vi "KrakenCommandPower.vi"(0 "Device Reference (in)":T1, 5 "Output Mode":T2(ring), 7 "Control Mode":enum16{"Safety", "Power"}(ring), 9 "Power or Testing Power":dbl, 11 "Error (in)":errorcluster) -> ()   [LabVIEW 2023]
doc: "Wrapper for commanding the power of a Talon FX motor controller. Supports voltage and safety interlock. Also supports the standard actuator testing interface and and the only sending new values on change."
uses:
  <vilib>/Rock Robotics/WPI/ThirdParty/Phoenix6/DeviceReference.ctl
  <vilib>/Rock Robotics/WPI/ThirdParty/Phoenix6/controls/DutyCycleOut SetControl.vi
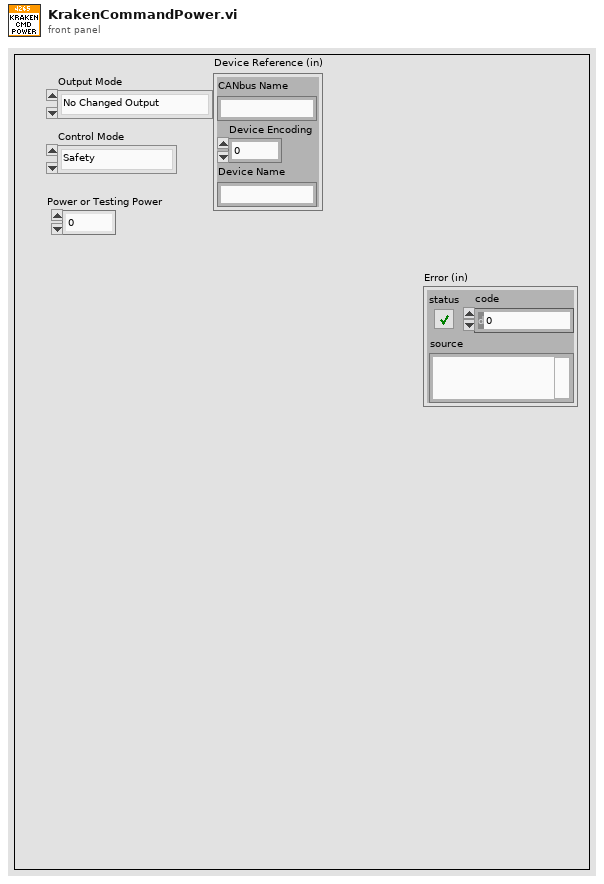
[diagram p1: front panel]
types:
  T1 = typedef "DeviceReference.ctl" = cluster{"CANbus Name":string, "Device Encoding":u32, "Device Name":string}
  T2 = enum16{"No Changed Output", "New Normal Output", "New Testing Output"}
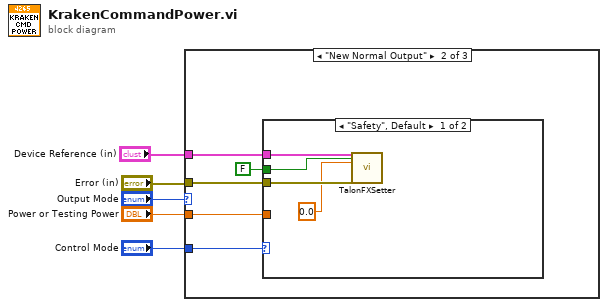
[diagram p0: block diagram]
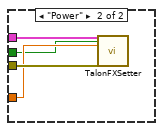
[diagram p3: hidden frame]
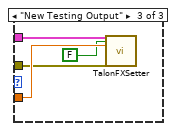
[diagram p4: hidden frame]
diagram:
  n1 = case shown="\"New Normal Output\"" "Output Mode" {
    tunnel: "Power or Testing Power" -> [_ w7 w22]
    tunnel: "Device Reference (in)" -> [_ w10 w20]
    tunnel: "Control Mode" -> [_ w9 _]
    tunnel: "Error (in)" -> [_ w8 w21]
    frame "No Changed Output", Default {
    }
    frame "New Normal Output" {
      n2 = case shown="\"Safety\", Default" w9 {
        tunnel: w10 -> [w13 w18]
        tunnel: w7 -> [_ w16]
        tunnel: w8 -> [w14 w17]
        tunnel: FALSE ("StopSendingOtherRequests") -> [w11 w15]
        frame "Safety", Default {
          n3 = call-poly <vilib>:"TalonFXSetter.vi"("DeviceReference"=w13, "StopSendingOtherRequests"=w11, "Output"=0.0, "error in"=w14) -> ()  [unwired: 22 in, 2 out]
        }
        frame "Power" {
          n4 = call-poly <vilib>:"TalonFXSetter.vi"("DeviceReference"=w18, "StopSendingOtherRequests"=w15, "Output"=w16, "error in"=w17) -> ()  [unwired: 22 in, 2 out]
        }
      }
    }
    frame "New Testing Output" {
      n5 = call-poly <vilib>:"TalonFXSetter.vi"("DeviceReference"=w20, "StopSendingOtherRequests"=FALSE, "Output"=w22, "error in"=w21) -> ()  [unwired: 22 in, 2 out]
    }
  }
